vi "MultiAI_Init.vi"(0 "channel list":string, 1 "error in":errorcluster) -> (2 "task out":refnum<k21>, 3 "(DAQ missing?)":bool caption="Initialization Problem", 4 "error out":errorcluster)   [LabVIEW 2015]
doc: "Sets up and starts a DAQmx task (named SimpleAI) to read multiple Analog inputs. The inputs will be in Referenced Single Ended mode, with an expected range of -10V to +10V. More than one input can be sampled simultaneously by wiring a comma separated list of channels to the \"channel list\" input, e.g. \"Dev1/ai0,Dev1/ai1\"."
uses:
  <vilib>/DAQmx/create/channels.llb/DAQmx Create Channel (AI-Voltage-Basic).vi
panel:
  # "Created by Dr. J. G. McLean\nand E. M . Pogozelski\nSUNY Geneseo      2006"
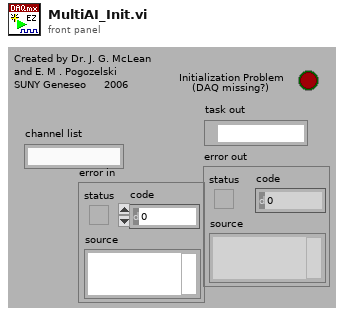
[diagram p1: front panel]
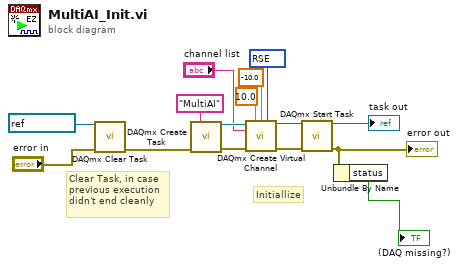
[diagram p0: block diagram]
diagram:
  w11 = 10083 items=["default"=-1, "differential"=10106, "RSE"=10083, "NRSE"=10078] ("input terminal configuration")
  # "Initiallize"
  # "Clear Task, in case\nprevious execution\ndidn't end cleanly"
  n1 = call <vilib>:"DAQmx Clear Task.vi"("task in"=refnum<k21> "MultiAI", "error in"="error in") -> ("error out"=w5:errorcluster)  [unwired: 13 in]
  n2 = call <vilib>:"DAQmx Create Task.vi"("new task name"="MultiAI", "error in"=w5) -> ("task out"=w14:refnum<k21>, "error out"=w10:errorcluster)  [unwired: 12 in]
  n3 = call-poly <vilib>:"DAQmx Create Virtual Channel.vi"("task in"=w14, "maximum value"=10.0, "minimum value"=-10.0, "input terminal configuration"=w11, "physical channels"="channel list", "error in"=w10) -> ("task out"=w9:refnum<k21>, "error out"=w8:errorcluster)  [unwired: 8 in]
  n4 = call <vilib>:"DAQmx Start Task.vi"("task/channels in"=w9, "error in"=w8) -> ("task out"=→"task out":refnum<k21>, "error out"=w6:errorcluster)  [unwired: 12 in]
  "error out" <- w6
  n5 = Unbundle By Name(w6) -> ("status"=→"(DAQ missing?)":bool)
